vi "LEDs.vi"   [LabVIEW 2019]
uses:
  Globals/LED_Globals.vi
  LED_States.ctl
  Globals/Flywheel_Globals.vi
  Globals/Intake_Globals.vi
types:
  T1 = typedef "CTRE_CANifier_DeviceRef.ctl" = cluster{"DeviceStatus":errorcluster, "Device Number":u8, "Handle":u64, "UsageFrame":u32, "Library Path":path}
  T2 = typedef "LED_States.ctl" = enum16{"Off", "Red", "Green", "Blinking Green", "Rainbow", "White"}
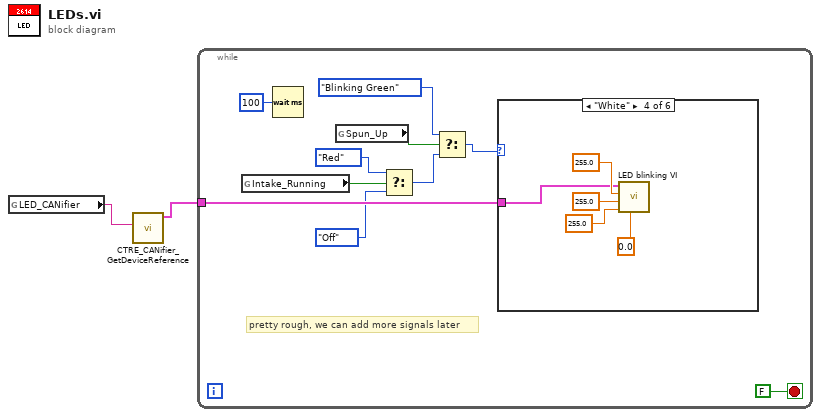
[diagram p0: block diagram]
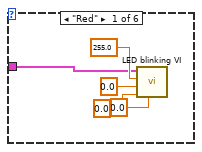
[diagram p2: hidden frame]
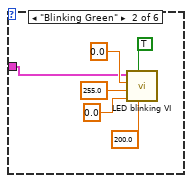
[diagram p3: hidden frame]
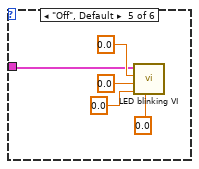
[diagram p5: hidden frame]
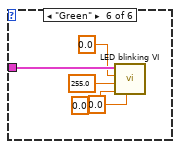
[diagram p6: hidden frame]
diagram:
  n1 = global read "LED_Globals.vi" "LED_CANifier"() -> (w1:string)
  n2 = call <vilib>:"CTRE_CANifier_GetDeviceReference.vi"("refnum name"=w1) -> ("CANifierDevRef"=w2:T1)  [unwired: 9 in, 1 out]
  n3 = while {
    tunnel: w2 -> [w10]
    stop <- FALSE stop-if-true
    # "pretty rough, we can add more signals later"
    n4 = global read "Intake_Globals.vi" "Intake_Running"() -> (w6:bool)
    n5 = Wait (ms)(milliseconds to wait=u32 100) -> ()  [unwired: 1 out]
    n6 = global read "Flywheel_Globals.vi" "Spun_Up"() -> (w7:bool)
    n7 = Select(t=LED_States."Red", s=w6, f=LED_States."Off") -> (s? t:f=w5:T2)
    n8 = Select(t=LED_States."Blinking Green", s=w7, f=w5) -> (s? t:f=w8:T2)
    n9 = case shown="\"White\"" w8 {
      tunnel: w10 -> [w14 w19 _ w24 w30 w38]
      frame "Red" {
        n10 = call "LED blinking VI.vi"("Wait time(ms)"=0.0 ("Wait time"), "Blue"=0.0, "Green"=0.0, "Red"=255.0, "CANifierDevRef"=w14) -> ()  [unwired: 7 in]
      }
      frame "Blinking Green" {
        n11 = call "LED blinking VI.vi"("Wait time(ms)"=200.0 ("Wait time"), "Blinking/not blinking"=TRUE, "Blue"=0.0, "Green"=255.0, "Red"=0.0, "CANifierDevRef"=w19) -> ()  [unwired: 6 in]
      }
      frame "Rainbow" {
        # "implement later"
      }
      frame "White" {
        n12 = call "LED blinking VI.vi"("Wait time(ms)"=0.0 ("Wait time"), "Blue"=255.0, "Green"=255.0, "Red"=255.0, "CANifierDevRef"=w24) -> ()  [unwired: 7 in]
      }
      frame "Off", Default {
        n13 = call "LED blinking VI.vi"("Wait time(ms)"=0.0 ("Wait time"), "Blue"=0.0, "Green"=0.0, "Red"=0.0, "CANifierDevRef"=w30) -> ()  [unwired: 7 in]
      }
      frame "Green" {
        n14 = call "LED blinking VI.vi"("Wait time(ms)"=0.0 ("Wait time"), "Blue"=0.0, "Green"=255.0, "Red"=0.0, "CANifierDevRef"=w38) -> ()  [unwired: 7 in]
      }
    }
  }
